vi "Stop Core.vi"(10 "final error code":i32, 11 "PS Control Actor in":refnum<class "PS Control Actor.lvclass">) -> (3 "PS Control Actor out":refnum<class "PS Control Actor.lvclass">)   [LabVIEW 2025, in "PS Control Actor.lvlib" / "PS Control Actor.lvclass"]
doc: "(<B>Filename</B>: Actor Framework.lvlib:Actor.lvclass:Stop Core.vi)\n\nDefines what the actor does before it stops. Use the <B>final error code</B> input to determine whether the actor shut down in response to an error.\n\nBy default, this method does nothing. A descendant class may override it to define behavior, such as shutting down any processes the actor initiated in its override of the Actor Core method.\nAuthor: Scott Hannahs <sth@magnet.fsu.edu>\n\nThis software is licensed for use under the “MIT License\"\nCopyright (c) 2025 Scott Hannahs, sth@sth@magnet.sthnet.net\n\nPermission is hereby granted, free of charge, to any person obtaining a copy of this software and associated documentation files (the \"Software\"), to deal in the Software without restriction, including without limitation the rights to use, copy, modify, merge, publish, distribute, sublicense, and/or sell copies of the Software, and to permit persons to whom the Software is furnished to do so, subject to the following conditions: The above copyright notice and this permission notice shall be included in all copies or substantial portions of the Software.\n\nTHE SOFTWARE IS PROVIDED \"AS IS\", WITHOUT WARRANTY OF ANY KIND, EXPRESS OR IMPLIED, INCLUDING BUT NOT LIMITED TO THE WARRANTIES OF MERCHANTABILITY, FITNESS FOR A PARTICULAR PURPOSE AND NONINFRINGEMENT. IN NO EVENT SHALL THE AUTHORS OR COPYRIGHT HOLDERS BE LIABLE FOR ANY CLAIM, DAMAGES OR OTHER LIABILITY, WHETHER IN AN ACTION OF CONTRACT, TORT OR OTHERWISE, ARISING FROM, OUT OF OR IN CONNECTION WITH THE SOFTWARE OR THE USE OR OTHER DEALINGS IN THE SOFTWARE."
uses:
  PS Control Actor.lvclass
  PS Control Actor.lvclass/PS Control Actor.ctl
  PS Driver/PS Driver.lvclass
  <vilib>/ActorFramework/Actor/Actor.lvclass
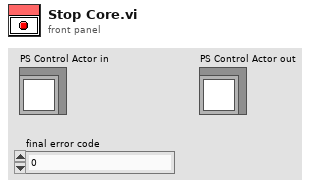
[diagram p1: front panel]
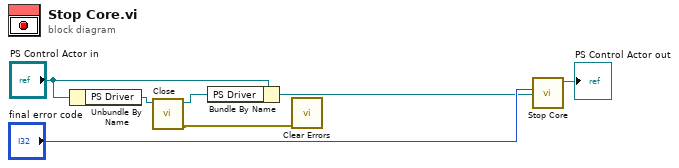
[diagram p0: block diagram]
diagram:
  n1 = Unbundle By Name("PS Control Actor in") -> ("PS Driver"=w2:refnum<class "PS Driver.lvclass">)
  n2 = call-dynamic "Close.vi"("PS Driver Actor in"=w2) -> ("error out"=w1:errorcluster, "PS Driver Actor out"=w3:refnum<class "PS Driver.lvclass">)  [unwired: 9 in]
  n3 = Bundle By Name(cluster="PS Control Actor in", "PS Driver"=w3) -> (w4:refnum<class "PS Control Actor.lvclass">)
  n4 = call <vilib>:"Clear Errors.vi"("error in (no error)"=w1) -> ()  [unwired: 5 in, 2 out]
  n5 = call-parent "Stop Core.vi"("final error code"="final error code", "Actor in"=w4) -> ("Actor out"=→"PS Control Actor out":refnum<class "PS Control Actor.lvclass">)  [unwired: 9 in]
